vi "Read ErrorData.vi"(8 "error in (no error)":errorcluster, 11 "Error in":refnum<class "Error.lvclass">) -> (0 "error out":errorcluster, 2 "ErrorData":T2, 3 "Error out":refnum<class "Error.lvclass">)   [LabVIEW 2019, in "Error.lvclass"]
uses:
  Error.lvclass
  TypeDef/Error Classification.ctl
  Error.lvclass/Error.ctl
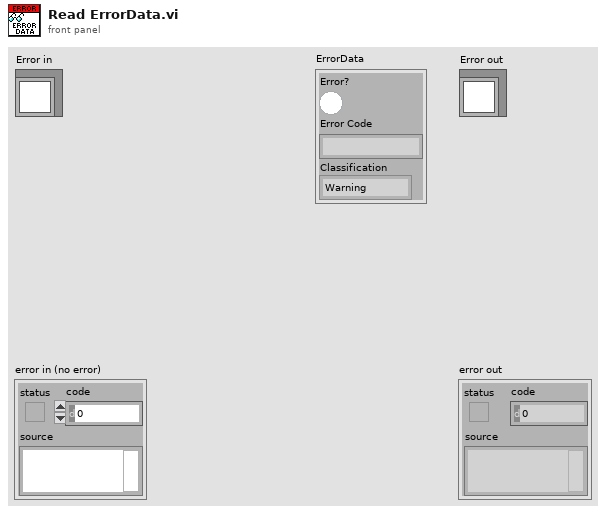
[diagram p1: front panel]
types:
  T1 = typedef "Error.lvclass/Error Classification.ctl" = enum16{"Warning"}
  T2 = cluster{"Error?":bool, "Error Code":string, "Classification":T1}
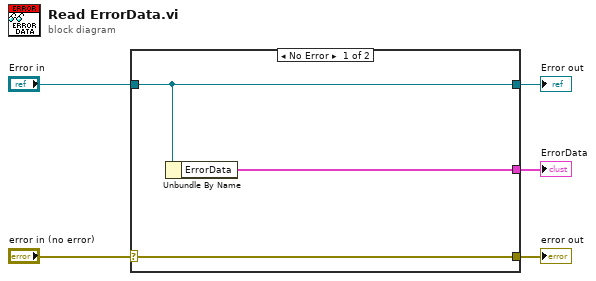
[diagram p0: block diagram]
diagram:
  n1 = case shown="No Error" "error in (no error)" {
    selector: "error in (no error)" -> [w8 w9]
    tunnel: [w8 w9] -> w4
    tunnel: [w7 w10] -> w2
    tunnel: "Error in" -> [w7 w10]
    tunnel: [w6 _] -> w1
    frame No Error {
      n2 = Unbundle By Name(w7) -> ("ErrorData"=w6:T2)
    }
    frame Error {
    }
  }
  "error out" <- w4
  "Error out" <- w2
  "ErrorData" <- w1
